vi "ALTS-2015 One Button Dialog Custom.vi"(8 "Error in":errorcluster, 11 "Message in":string="Test") -> (0 "Error out":errorcluster, 3 "OK?":bool)   [LabVIEW 2013]
panel:
  in  "OK?":bool caption="Start"
  out "Message Display":string
  out "Blink":bool
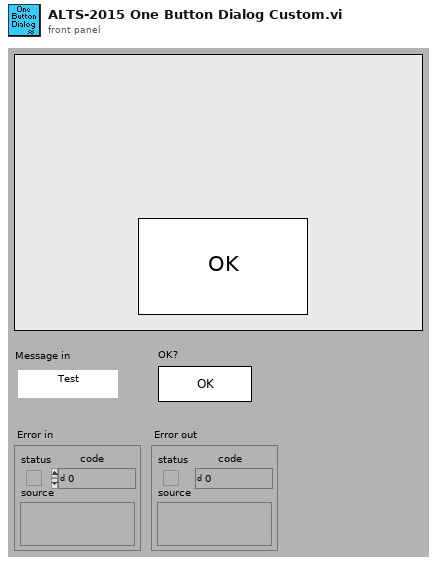
[diagram p1: front panel]
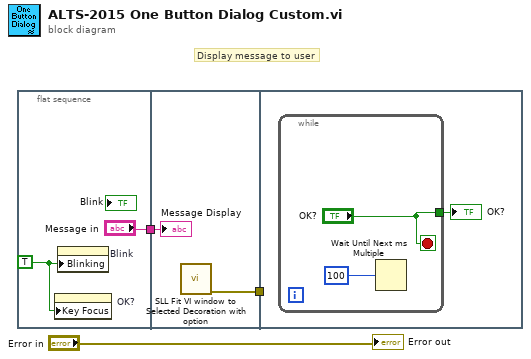
[diagram p0: block diagram]
diagram:
  # "Display message to user"
  n1 = flat-sequence {
    tunnel: ["Message in"] -> w2
    tunnel: w2 -> [w7]
    tunnel: [w6] -> w1
    tunnel: w1 -> [_]
    frame #0 {
      w4 = TRUE ("Blinking")
      n2 = property on="OK?" class="Bool"("Key Focus"=w4) -> ()  [unwired: 2 in, 2 out]
      n3 = property on="Blink" class="Bool"("Blinking"=w4) -> ()  [unwired: 2 in, 2 out]
    }
    frame #1 {
      n4 = call <userlib>:"SLL Fit VI window to Selected Decoration with option.vi"() -> ("error out"=w6:errorcluster)  [unwired: 10 in, 1 out]
      "Message Display" <- w7
    }
    frame #2 {
      n5 = while {
        tunnel: ["OK?"] -> w8
        stop <- "OK?" stop-if-true
        n6 = Wait Until Next ms Multiple(millisecond multiple=u32 100 ("milliseconds to wait")) -> ()  [unwired: 1 out]
      }
      "OK?" <- w8
    }
  }
  "Error out" <- "Error in"
